vi "FIFO Check boolean logic.vi"(9 "Elements Remaining":u32, 11 "Read at least":u32) -> (2 "Read FIFO":bool, 3 "No more data":bool)   [LabVIEW 2013]
panel:
  # "RE-ENTRANT"
  # "SUB-ROUTINE"
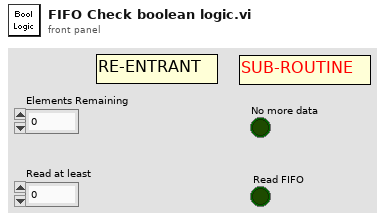
[diagram p1: front panel]
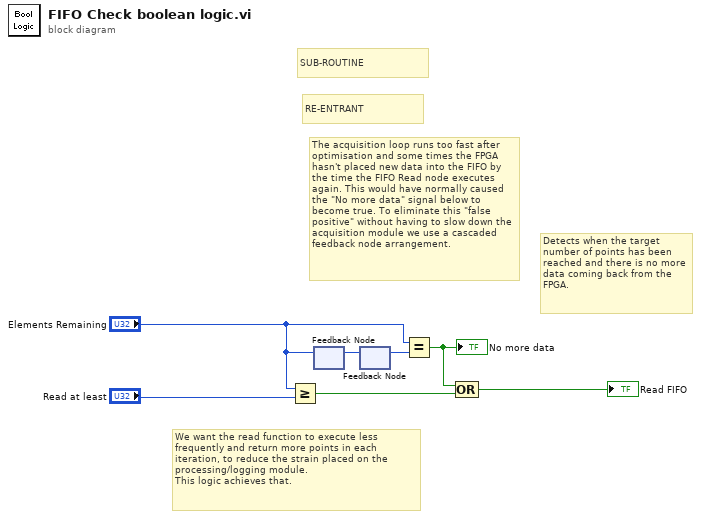
[diagram p0: block diagram]
diagram:
  # "SUB-ROUTINE"
  # "RE-ENTRANT"
  # "The acquisition loop runs too fast after optimisation and some times the FPGA hasn't placed new data into the FIFO by the time the FIFO Read node executes again. This would have normally caused the \"No more data\" signal below to become true. To eliminate this \"false positive\" without having to slow down the acquisition module we use a cascaded feedback node arrangement."
  # "Detects when the target number of points has been reached and there is no more data coming back from the FPGA."
  # "We want the read function to execute less frequently and return more points in each iteration, to reduce the strain placed on the processing/logging module.\nThis logic achieves that."
  n1 = Greater Or Equal?(x="Elements Remaining", y="Read at least") -> (x >= y?=w6:bool)
  n2 = feedback #1() -> (w2:u32)  [unwired: 1 in]
  n3 = feedback-in #1("Elements Remaining") -> ()
  n4 = feedback #2() -> (w3:u32)  [unwired: 1 in]
  n5 = feedback-in #2(w2) -> ()
  n6 = Equal?(x="Elements Remaining", y=w3) -> (x = y?=w5:bool)
  "No more data" <- w5
  n7 = Compound Arithmetic op=OR(w5, w6) -> (→"Read FIFO":bool)
